vi "live view D01.vi"() -> ()   [LabVIEW 2019, in "D01.lvlib"]
uses:
  D01.lvlib
  <vilib>/userDefined/High Color/IMAQdx.ctl
  <vilib>/vision/Image Controls.llb/IMAQ Image.ctl
  <vilib>/measure/mamon.llb/Trigger Detection for 1 Channel.vi
  <vilib>/measure/NI_MAPro.lvlib
  Calibration Lib.lvlib
  database.lvlib
  <vilib>/vision/driver/NI_Vision_Acquisition_Software.lvlib
panel:
  out "Error out":errorcluster
  in  "Save Button":bool
  in  "Calib IMQ Num":u16(ring) items=["First IMQ", "Second IMQ", "Third IMQ"]
  in  "Verify Calibration1 D01":bool caption="capture grab"
  in  "snapshot":bool
  out "error prj26":errorcluster
  in  "Verify Calibration D01":bool caption="capture grab"
  in  "Close":bool
  in  "Method 2 save D01":bool caption="capture grab"
  in  "Method 1 Save D01":bool caption="Saving txt"
  out "Average Result":string="Average Result"
  out ">16  A":dbl(slide)=1.0 caption=">16 mm" scale=0.0..100.0
  out "14-16  A":dbl(slide)=1.0 caption="14.16 mm" scale=0.0..100.0
  out "12.7-14 A":dbl(slide)=1.0 caption="12.7-14 mm" scale=0.0..100.0
  out "11-12.7 A":dbl(slide)=1.0 caption="11-12.7 mm" scale=0.0..100.0
  out "9.5-11  A":dbl(slide)=1.0 caption="9.5-11 mm" scale=0.0..100.0 scale format="%#_4f"
  out "8-9.5  A":dbl(slide)=1.0 caption="8-9.5 mm" scale=0.0..100.0
  out "6.3-8  A":dbl(slide)=1.0 caption="6.3-8 mm" scale=0.0..100.0
  out "<6.3  A":dbl(slide)=1.0 caption="<6.3 mm" scale=0.0..100.0
  out "Live Result":string="Live Result"
  out ">16  L":dbl(slide)=1.0 caption=">16 mm" scale=0.0..100.0
  out "Live View":T1(plugin-control) caption="Disc 26"
  out "14-16  L":dbl(slide)=1.0 caption="14-16 mm" scale=0.0..100.0
  out "12.7-14  L":dbl(slide)=1.0 caption="12.7-14 mm" scale=0.0..100.0
  out "11-12.7L":dbl(slide)=1.0 caption="11-12.7 mm" scale=0.0..100.0
  out "9.5-11  L":dbl(slide)=1.0 caption="9.5-11 mm" scale=0.0..100.0 scale format="%#_4f"
  out "8-9.5  L":dbl(slide)=1.0 caption="8-9.5 mm" scale=0.0..100.0
  out "6.3-8  L":dbl(slide)=1.0 caption="6.3-8 mm" scale=0.0..100.0
  out "<6.3  L":dbl(slide)=1.0 caption="<6.3 mm" scale=0.0..100.0
  out "disc name":string="Live Info Disc 01"
  out "dsgs":string="DSGS"
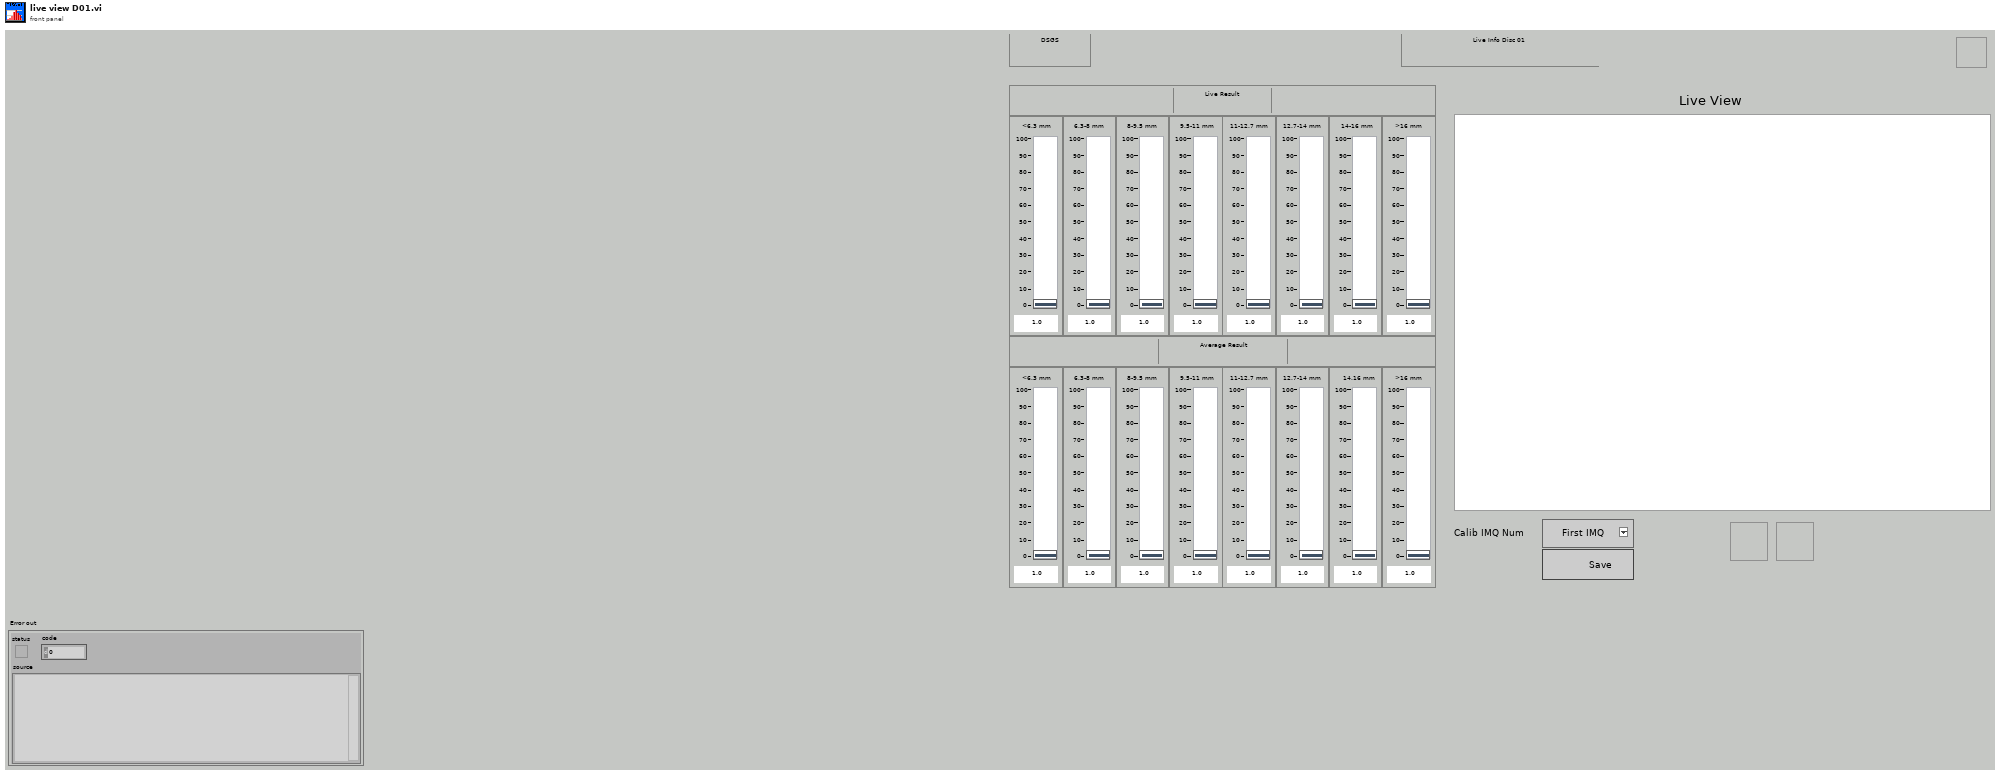
[diagram p1: front panel]
types:
  T1 = typedef "IMAQ Image.ctl" = refnum<image>
  T2 = typedef "IMAQdx.ctl" = refnum<k21>
  T3 = enum8{"Enabled", "Disabled", "Disabled and Grayed Out"}
  T4 = cluster{"date/time string":string, "date/time string":string, string, "Value":dbl, "Value":dbl, "Value":dbl, "Value":dbl, "Value":dbl, "Value":dbl, "Value":dbl, "Value":dbl}
  T5 = cluster{"date/time string":string, "date/time string":string, i32, "spreadsheet string":string, "spreadsheet string":string}
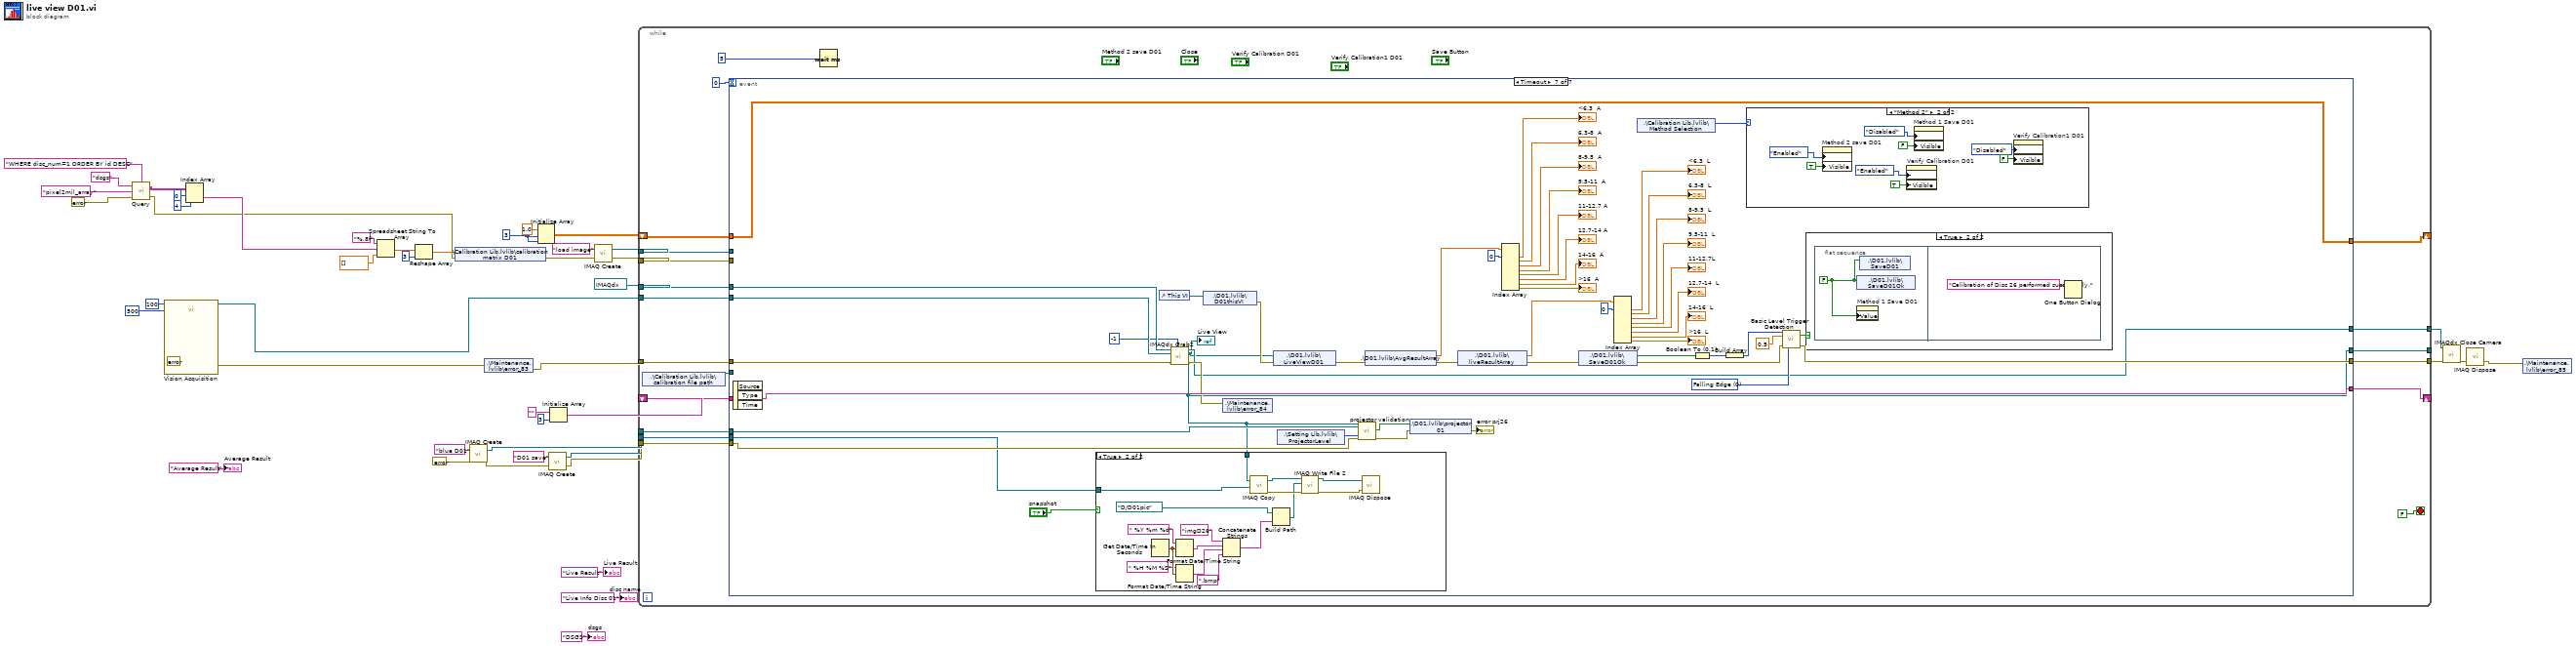
[diagram p0: block diagram]
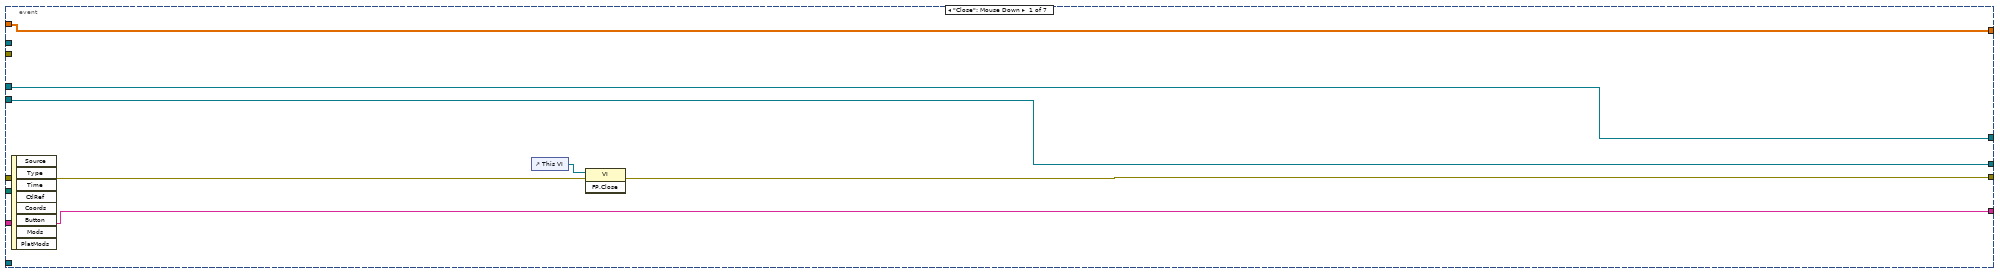
[diagram p2: hidden frame]
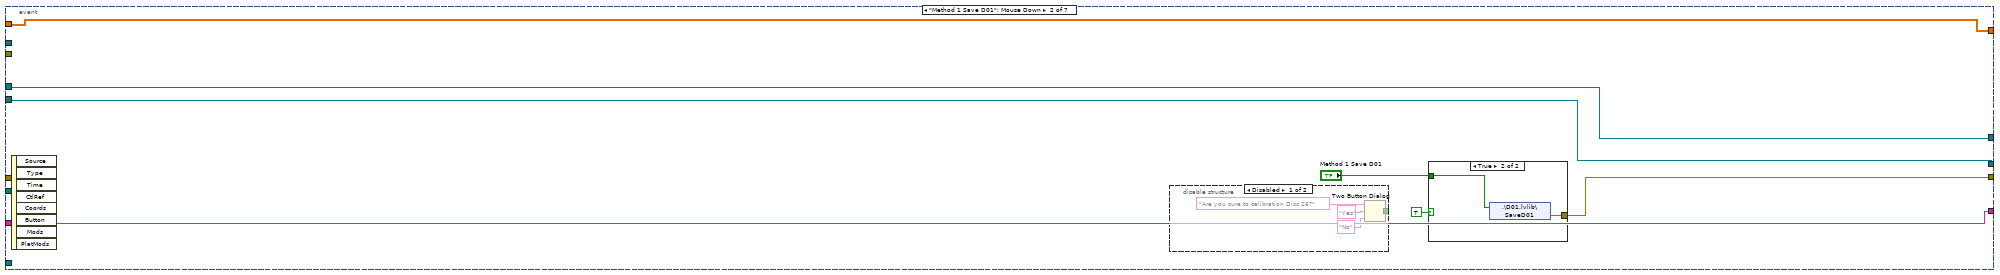
[diagram p3: hidden frame]
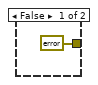
[diagram p5: hidden frame]
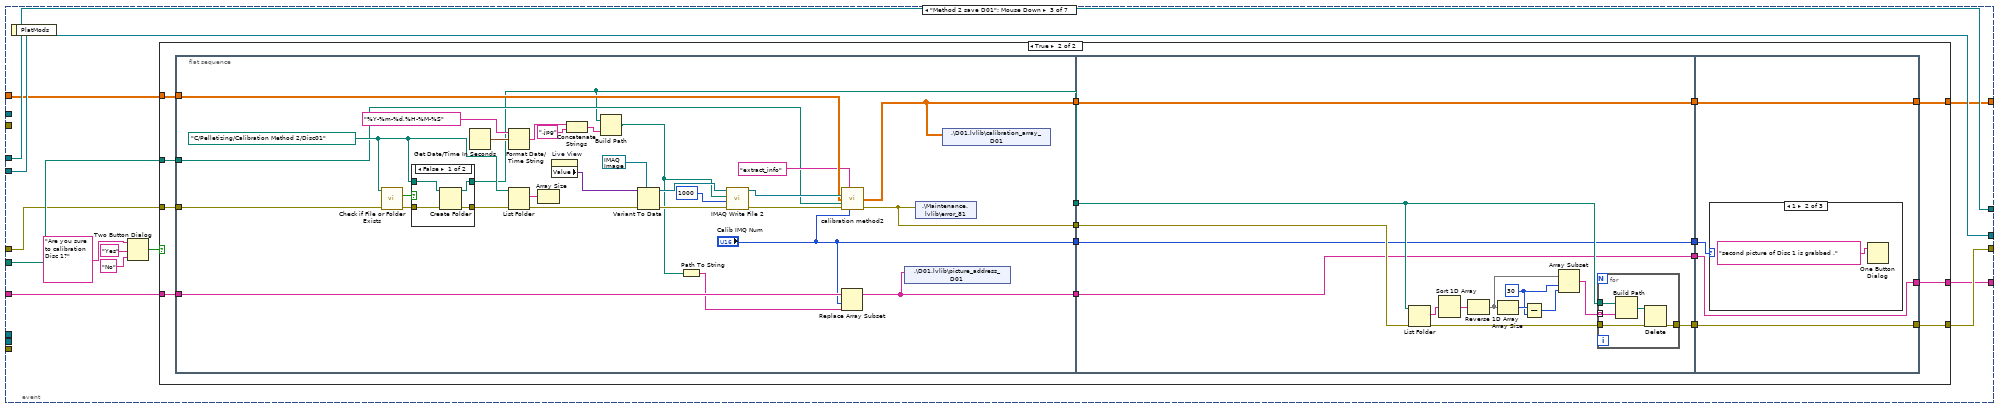
[diagram p6: hidden frame]
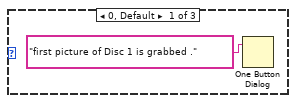
[diagram p9: hidden frame]
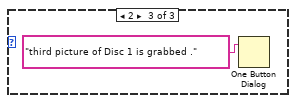
[diagram p10: hidden frame]
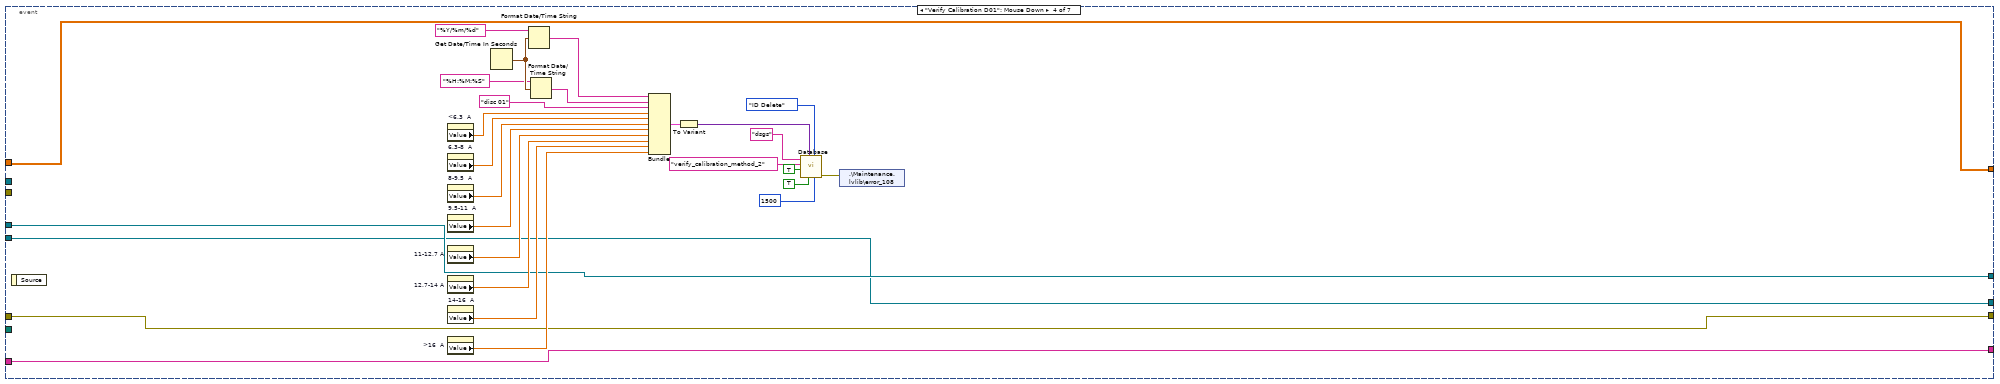
[diagram p11: hidden frame]
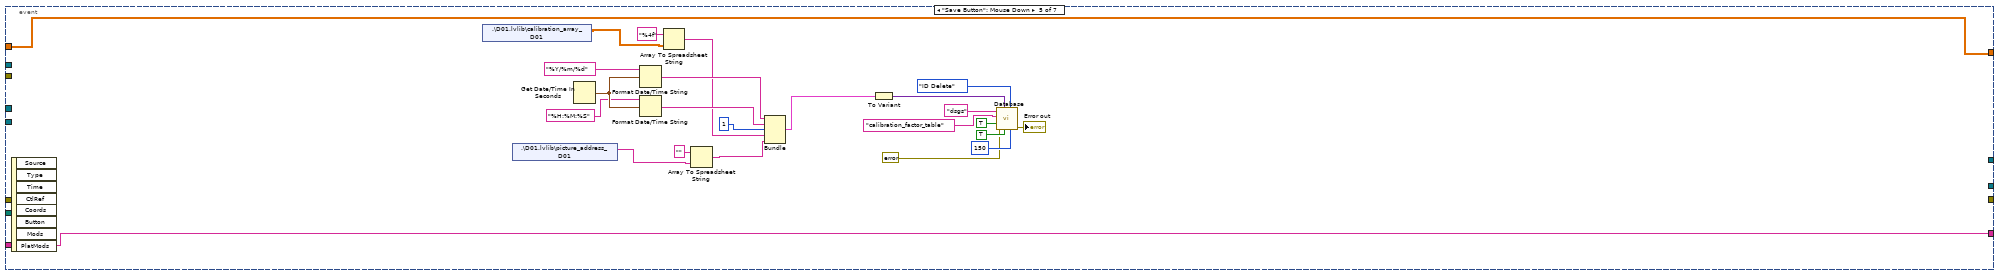
[diagram p12: hidden frame]
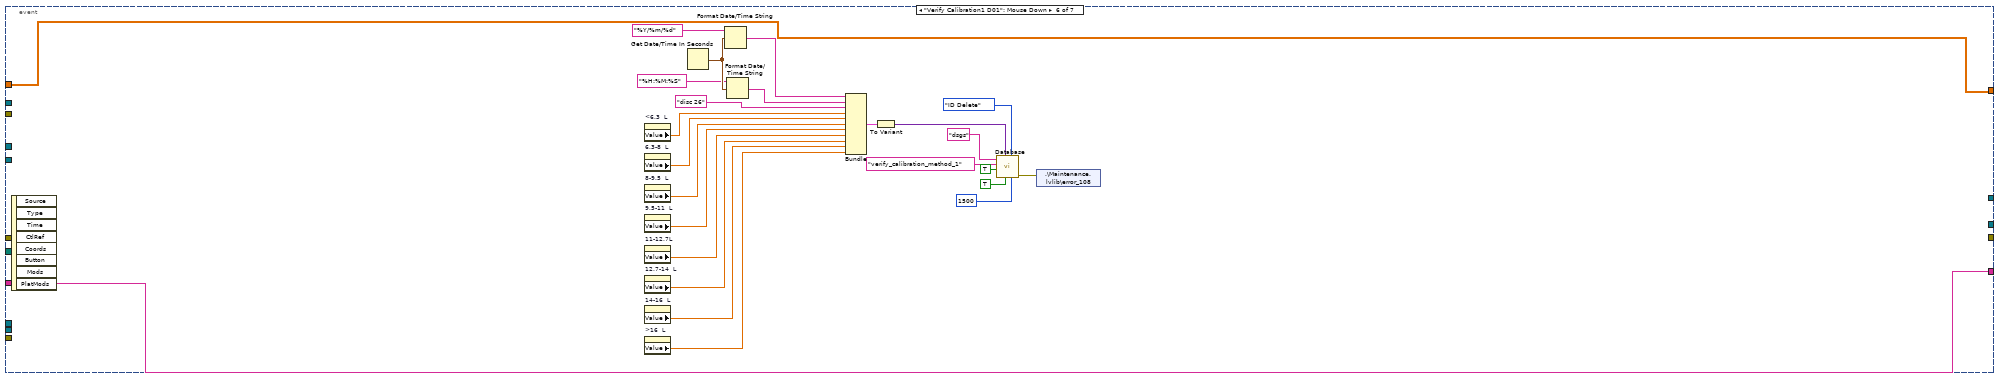
[diagram p13: hidden frame]
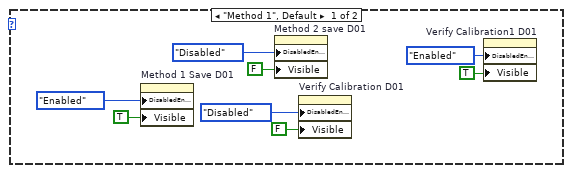
[diagram p15: hidden frame]
diagram:
  w15 = 3 ("dimension size")
  (unwired) errorcluster {"status"=FALSE, "code"=0, "source"=""} ("error in (no error)")
  n1 = call "Query.vi"("Condition"="WHERE disc_num=1 ORDER BY id DESC", "Error in"=errorcluster {"status"=FALSE, "code"=0, "source"=""}, "Table Name"="pixel2mil_array", "Connection Name"="dsgs") -> ("Error out"=w7:errorcluster, "data"=w10:string[][])
  n2 = call "Vision Acquisition"("Gain (Raw)"=i64 100, "Exposure Time (Raw)"=i64 500) -> ("Image Out"=w4:T1, "error out"=w3:errorcluster)  [unwired: 23 in, 1 out]
  n3 = Index Array(array=w10, index (row)=0, index (col)=4 ("disabled index (col)")) -> (element=w8:string)
  n4 = Spreadsheet String To Array(format string="%.8f", spreadsheet string=w8, array type (2D Dbl)=sgl[] []) -> (array=w28:sgl[])  [unwired: 1 in]
  n5 = Reshape Array(w28, 3 ("dimension size")) -> (w25:sgl[])
  n6 = shared-variable ".\\Calibration Lib.lvlib\\calibration matrix D01"(w25, error in=w7) -> (error out=w24:errorcluster)
  n7 = call "IMAQ Create"("Image Name"="blue D01", "error in (no error)"=errorcluster {"status"=FALSE, "code"=0, "source"=""}) -> ("New Image"=w22:T1, "error out"=w20:errorcluster)  [unwired: 3 in]
  n8 = shared-variable ".\\Maintenance.lvlib\\error_83"(w3) -> (error out=w37:errorcluster)  [unwired: 1 in]
  n9 = Initialize Array(1.0 ("element"), w15, w15) -> (w14:dbl[][])
  n10 = call "IMAQ Create"("Image Name"="D01 save", "error in (no error)"=w20) -> ("New Image"=w17:T1, "error out"=w19:errorcluster)  [unwired: 3 in]
  n11 = Initialize Array("", 3 ("dimension size")) -> (w11:string[])
  n12 = call "IMAQ Create"("Image Name"="load image", "error in (no error)"=w24) -> ("New Image"=w34:T1, "error out"=w35:errorcluster)  [unwired: 3 in]
  n13 = while {
    tunnel: w37 -> [w62]
    tunnel: w4 -> [w60]
    tunnel: [w59] -> w41
    tunnel: [w58] -> _
    tunnel: T2 "cam0" ("Session In") -> [w57]
    tunnel: [w56] -> w38
    tunnel: w35 -> [w55]
    tunnel: w34 -> [w54]
    tunnel: w22 -> [w53]
    tunnel: w19 -> [w52]
    tunnel: w17 -> [w51]
    shift-right: [w49] -> _
    shift-left: w14 -> [w50]
    shift-right: [w47] -> _
    shift-left: w11 -> [w48]
    stop <- FALSE stop-if-true
    n14 = shared-variable ".\\Calibration Lib.lvlib\\calibration file path"() -> (w46:path)  [unwired: 1 in, 1 out]
    n15 = event shown="[6] Timeout" {
      selector: _ -> [_ _ _ _ _ _ _]
      dyn-events: _ -> [_ _ _ _ _ _ _]
      timeout: 0 -> [_ _ _ _ _ _ _]
      tunnel: w46 -> [_ _ w98 _ _ _ _]
      tunnel: [w70 w78 w94 w186 _ _ w275] -> w59
      tunnel: w62 -> [w69 _ w97 w186 _ _ w263]
      tunnel: w60 -> [w68 w77 w96 w184 _ _ w261]
      tunnel: [w68 w77 w96 w184 _ _ w257] -> w58
      tunnel: w57 -> [w67 w76 w95 w185 _ _ w260]
      tunnel: [w67 w76 w95 w185 _ _ w258] -> w56
      tunnel: w55 -> [_ _ _ _ _ _ _]
      tunnel: w54 -> [_ _ _ _ _ _ _]
      tunnel: w53 -> [_ _ _ _ _ _ w273]
      tunnel: w52 -> [_ _ _ _ _ _ w269]
      tunnel: w51 -> [_ _ _ _ _ _ w266]
      tunnel: w50 -> [w66 w73 w89 w181 w210 w233 w265]
      tunnel: [w66 w73 w88 w181 w210 w233 w265] -> w49
      tunnel: w48 -> [w65 w72 w87 w180 w209 w232 w264]
      tunnel: [w65 w72 w86 w180 w209 w232 w264] -> w47
      event "Close": Mouse Down {
        n16 = event-data() -> ()  [unwired: 1 in, 8 out]
        n17 = control-ref of="This VI"() -> (w71:refnum<vi>)
        n18 = invoke class="VI" method="FP.Close"(reference=w71, error in=w69) -> (error out=w70:errorcluster)  [unwired: 1 in, 2 out]
      }
      event "Method 1 Save D01": Mouse Down {
        n19 = event-data() -> ()  [unwired: 1 in, 8 out]
        n20 = disable-structure shown="Disabled" {
          disable-tunnel: [w79 _] -> _
          frame Disabled {
            n21 = Two Button Dialog(message="Are you sure to calibration Disc 26?", 1:"No" ("F button name (\"Cancel\")"), 2:"Yes" ("T button name (\"OK\")")) -> (T button?=w79:bool)
          }
          frame Enabled {
          }
        }
        n22 = case shown="True" TRUE {
          tunnel: [errorcluster {"status"=FALSE, "code"=0, "source"=""} ("error IO") w85] -> w78
          tunnel: "Method 1 Save D01" -> [_ w84]
          frame False {
          }
          frame True {
            n23 = shared-variable ".\\D01.lvlib\\SaveD01"(w84) -> (error out=w85:errorcluster)  [unwired: 1 in]
          }
        }
      }
      event "Method 2 save D01": Mouse Down {
        n24 = event-data() -> ()  [unwired: 1 in, 1 out]
        n25 = Two Button Dialog(message="Are you sure to calibration Disc 1?", 1:"No" ("F button name (\"Cancel\")"), 2:"Yes" ("T button name (\"OK\")")) -> (T button?=w90:bool)
        n26 = case shown="True" w90 {
          tunnel: w98 -> [_ w116]
          tunnel: w97 -> [w101 w115]
          tunnel: [w101 w114] -> w94
          tunnel: w89 -> [w100 w112]
          tunnel: [w100 w109] -> w88
          tunnel: w87 -> [w99 w108]
          tunnel: [w99 w105] -> w86
          frame False {
          }
          frame True {
            n27 = flat-sequence {
              tunnel: w115 -> [w137]
              tunnel: w116 -> [w122]
              tunnel: [w118] -> w117
              tunnel: w112 -> [w130]
              tunnel: [w129] -> w110
              tunnel: w108 -> [w126]
              tunnel: [w125] -> w106
              tunnel: [w124] -> w104
              tunnel: ["Calib IMQ Num"] -> w102
              tunnel: [w158] -> w113
              tunnel: [w156] -> w111
              tunnel: [w155] -> w107
              tunnel: [w154] -> w103
              tunnel: w102 -> [w154]
              tunnel: w104 -> [w159]
              tunnel: w106 -> [w155]
              tunnel: w110 -> [w156]
              tunnel: w117 -> [w160]
              tunnel: [w176] -> w114
              tunnel: w113 -> [w176]
              tunnel: [w175] -> w109
              tunnel: w111 -> [w175]
              tunnel: [w174] -> w105
              tunnel: w107 -> [w174]
              tunnel: w103 -> [w173]
              frame #0 {
                w133 = path "C:/Pelletizing/Calibration Method 2/Disc01" ("path")
                n28 = call <vilib>:"Check if File or Folder Exists.vi"("error in (no error)"=w137, "path"=w133) -> ("error out"=w138:errorcluster, "file or folder exists?"=w139:bool)  [unwired: 7 in, 1 out]
                n29 = case shown="False" w139 {
                  tunnel: [w149 w153] -> w118
                  tunnel: w133 -> [w151 w153]
                  tunnel: w138 -> [w150 w152]
                  tunnel: [w148 w152] -> w135
                  frame False {
                    n30 = Create Folder(path (use dialog)=w151, error in=w150) -> (created path=w149:path, error out=w148:errorcluster)  [unwired: 1 in, 1 out]
                  }
                  frame True {
                  }
                }
                n31 = Get Date/Time In Seconds() -> (seconds since 1Jan1904=w143:timestamp)
                n32 = Format Date/Time String(time format string (%c)="%Y-%m-%d,%H-%M-%S", seconds (now)=w143) -> (date/time string=w141:string)  [unwired: 1 in]
                n33 = List Folder(path=w133, error in=w135) -> (filenames=w136:string[], error out=w134:errorcluster)  [unwired: 2 in, 2 out]
                n34 = Array Size(array=w136) -> ()  [unwired: 1 out]
                n35 = property on="Live View" class="ImageControl"() -> ("Value"=w147:variant)  [unwired: 2 in, 2 out]
                n36 = Concatenate Strings(w141, ".jpg" ("string")) -> (w121:string)
                n37 = Build Path(base path=w118, name or relative path=w121) -> (appended path=w120:path)
                n38 = Variant To Data(error in=w134, type=T1 refnum ("New Image"), Variant=w147) -> (data=w131:T1, error out=w144:errorcluster)
                n39 = Path To String(path=w120) -> (string=w119:string)
                n40 = call-poly "IMAQ Write File 2"("error in (no error)"=w144, "Image Quality"=u32 1000, "File Path"=w120, "Image"=w131) -> ("error out"=w128:errorcluster, "Image Out (duplicate)"=w132:T1)  [unwired: 6 in]
                n41 = Replace Array Subset(array=w126, new element=w119, index="Calib IMQ Num") -> (w125:string[])
                n42 = call "calibration method2.vi"("function name"="extract_info", "Image IN"=w132, "initialize matrix"=w130, "module path"=w122, "error in"=w128, "snap number"="Calib IMQ Num") -> ("calibration matrix"=w129:dbl[][], "error out"=w124:errorcluster)  [unwired: 8 in]
                n43 = shared-variable ".\\D01.lvlib\\picture_address_D01"(w125) -> ()  [unwired: 1 in, 1 out]
                n44 = shared-variable ".\\Maintenance.lvlib\\error_81"(w124) -> ()  [unwired: 1 in, 1 out]
                n45 = shared-variable ".\\D01.lvlib\\calibration_array_D01"(w129) -> ()  [unwired: 1 in, 1 out]
              }
              frame #1 {
                w161 = 30 ("index")
                n46 = List Folder(path=w160, error in=w159) -> (filenames=w167:string[], error out=w157:errorcluster)  [unwired: 2 in, 2 out]
                n47 = Sort 1D Array(array=w167) -> (sorted array=w166:string[])
                n48 = Reverse 1D Array(array=w166) -> (reversed array=w165:string[])
                n49 = Array Size(array=w165) -> (size(s)=w164:i32)
                n50 = Subtract(x=w164, y=w161) -> (x-y=w163:i32)
                n51 = Array Subset(array=w165, index=w161, length=w163) -> (w162:string[])
                n52 = for {
                  tunnel: w162 -> [w171] mode=indexing
                  tunnel: w160 -> [w172]
                  tunnel: [w169] -> w158
                  tunnel: w157 -> [w168]
                  n53 = Build Path(base path=w172, name or relative path=w171) -> (appended path=w170:path)
                  n54 = Delete(path (use dialog)=w170, error in=w168) -> (error out=w169:errorcluster)  [unwired: 3 in, 2 out]
                }
              }
              frame #2 {
                n55 = case shown="1" w173 {
                  frame 0, Default {
                    n56 = One Button Dialog(message="first picture of Disc 1 is grabbed .") -> ()  [unwired: 1 in, 1 out]
                  }
                  frame 1 {
                    n57 = One Button Dialog(message="second picture of Disc 1 is grabbed .") -> ()  [unwired: 1 in, 1 out]
                  }
                  frame 2 {
                    n58 = One Button Dialog(message="third picture of Disc 1 is grabbed .") -> ()  [unwired: 1 in, 1 out]
                  }
                }
              }
            }
          }
        }
      }
      event "Verify Calibration D01": Mouse Down {
        n59 = event-data() -> ()  [unwired: 1 in, 1 out]
        n60 = property on="<6.3  A" class="Slide (strict)"() -> ("Value"=w201:dbl)  [unwired: 2 in, 2 out]
        n61 = property on="6.3-8  A" class="Slide (strict)"() -> ("Value"=w200:dbl)  [unwired: 2 in, 2 out]
        n62 = property on="8-9.5  A" class="Slide (strict)"() -> ("Value"=w199:dbl)  [unwired: 2 in, 2 out]
        n63 = property on="9.5-11  A" class="Slide (strict)"() -> ("Value"=w198:dbl)  [unwired: 2 in, 2 out]
        n64 = property on="11-12.7 A" class="Slide (strict)"() -> ("Value"=w197:dbl)  [unwired: 2 in, 2 out]
        n65 = property on="12.7-14 A" class="Slide (strict)"() -> ("Value"=w196:dbl)  [unwired: 2 in, 2 out]
        n66 = property on="14-16  A" class="Slide (strict)"() -> ("Value"=w195:dbl)  [unwired: 2 in, 2 out]
        n67 = property on=">16  A" class="Slide (strict)"() -> ("Value"=w194:dbl)  [unwired: 2 in, 2 out]
        n68 = Get Date/Time In Seconds() -> (seconds since 1Jan1904=w206:timestamp)
        n69 = Format Date/Time String(time format string (%c)="%Y/%m/%d", seconds (now)=w206) -> (date/time string=w204:string)  [unwired: 1 in]
        n70 = Format Date/Time String(time format string (%c)="%H:%M:%S", seconds (now)=w206) -> (date/time string=w203:string)  [unwired: 1 in]
        n71 = Bundle("date/time string"=w204, "date/time string"=w203, "disc 01", "Value"=w201, "Value"=w200, "Value"=w199, "Value"=w198, "Value"=w197, "Value"=w196, "Value"=w195, "Value"=w194) -> (w193:T4)  [unwired: 1 in]
        n72 = To Variant(anything=w193) -> (Variant=w192:variant)
        n73 = call "Database.vi"("Maximum Row"=1500, "Enum"=enum16{"ID Delete", "Time Delete"}."ID Delete", "Delete row?"=TRUE, "Data"=w192, "Auto Increment ID?"=TRUE, "Table"="verify_calibration_method_2", "Connection"="dsgs") -> ("Error out"=w187:errorcluster)  [unwired: 4 in]
        n74 = shared-variable ".\\Maintenance.lvlib\\error_108"(w187) -> ()  [unwired: 1 in, 1 out]
      }
      event "Save Button": Mouse Down {
        n75 = event-data() -> ()  [unwired: 1 in, 8 out]
        n76 = shared-variable ".\\D01.lvlib\\calibration_array_D01"() -> (w211:dbl[][])  [unwired: 1 in, 1 out]
        n77 = shared-variable ".\\D01.lvlib\\picture_address_D01"() -> (w213:string[])  [unwired: 1 in, 1 out]
        n78 = Get Date/Time In Seconds() -> (seconds since 1Jan1904=w220:timestamp)
        n79 = Format Date/Time String(time format string (%c)="%Y/%m/%d", seconds (now)=w220) -> (date/time string=w221:string)  [unwired: 1 in]
        n80 = Format Date/Time String(time format string (%c)="%H:%M:%S", seconds (now)=w220) -> (date/time string=w219:string)  [unwired: 1 in]
        n81 = Array To Spreadsheet String(array=w211, 3:"%4f" ("format string")) -> (spreadsheet string=w215:string)  [unwired: 1 in]
        n82 = Array To Spreadsheet String(array=w213, 3:"" ("format string")) -> (spreadsheet string=w212:string)  [unwired: 1 in]
        n83 = Bundle("date/time string"=w221, "date/time string"=w219, 1, "spreadsheet string"=w215, "spreadsheet string"=w212) -> (w224:T5)  [unwired: 1 in]
        n84 = To Variant(anything=w224) -> (Variant=w231:variant)
        n85 = call "Database.vi"("Maximum Row"=150, "Enum"=enum16{"ID Delete", "Time Delete"}."ID Delete", "Delete row?"=TRUE, "Data"=w231, "Error in"=errorcluster {"status"=FALSE, "code"=0, "source"=""}, "Auto Increment ID?"=TRUE, "Table"="calibration_factor_table", "Connection"="dsgs") -> ("Error out"=→"Error out":errorcluster)  [unwired: 3 in]
      }
      event "Verify Calibration1 D01": Mouse Down {
        n86 = event-data() -> ()  [unwired: 1 in, 8 out]
        n87 = property on="<6.3  L" class="Slide (strict)"() -> ("Value"=w250:dbl)  [unwired: 2 in, 2 out]
        n88 = property on="6.3-8  L" class="Slide (strict)"() -> ("Value"=w249:dbl)  [unwired: 2 in, 2 out]
        n89 = property on="8-9.5  L" class="Slide (strict)"() -> ("Value"=w248:dbl)  [unwired: 2 in, 2 out]
        n90 = property on="9.5-11  L" class="Slide (strict)"() -> ("Value"=w247:dbl)  [unwired: 2 in, 2 out]
        n91 = property on="11-12.7L" class="Slide (strict)"() -> ("Value"=w246:dbl)  [unwired: 2 in, 2 out]
        n92 = property on="12.7-14  L" class="Slide (strict)"() -> ("Value"=w245:dbl)  [unwired: 2 in, 2 out]
        n93 = property on="14-16  L" class="Slide (strict)"() -> ("Value"=w244:dbl)  [unwired: 2 in, 2 out]
        n94 = property on=">16  L" class="Slide (strict)"() -> ("Value"=w243:dbl)  [unwired: 2 in, 2 out]
        n95 = Get Date/Time In Seconds() -> (seconds since 1Jan1904=w255:timestamp)
        n96 = Format Date/Time String(time format string (%c)="%Y/%m/%d", seconds (now)=w255) -> (date/time string=w253:string)  [unwired: 1 in]
        n97 = Format Date/Time String(time format string (%c)="%H:%M:%S", seconds (now)=w255) -> (date/time string=w252:string)  [unwired: 1 in]
        n98 = Bundle("date/time string"=w253, "date/time string"=w252, "disc 26", "Value"=w250, "Value"=w249, "Value"=w248, "Value"=w247, "Value"=w246, "Value"=w245, "Value"=w244, "Value"=w243) -> (w242:T4)  [unwired: 1 in]
        n99 = To Variant(anything=w242) -> (Variant=w241:variant)
        n100 = call "Database.vi"("Maximum Row"=1500, "Enum"=enum16{"ID Delete", "Time Delete"}."ID Delete", "Delete row?"=TRUE, "Data"=w241, "Auto Increment ID?"=TRUE, "Table"="verify_calibration_method_1", "Connection"="dsgs") -> ("Error out"=w236:errorcluster)  [unwired: 4 in]
        n101 = shared-variable ".\\Maintenance.lvlib\\error_108"(w236) -> ()  [unwired: 1 in, 1 out]
      }
      event Timeout {
        w283 = u16 0 items=["Falling Edge", "Rising Edge"] ("trigger slope")
        n102 = event-data() -> ()  [unwired: 1 in, 3 out]
        n103 = control-ref of="This VI"() -> (w278:refnum<vi>)
        n104 = call <vilib>:"IMAQdx Grab2.vi"("Timeout (ms)"=-1, "error in"=w263, "Image In"=w261, "Session In"=w260) -> ("error out"=w262:errorcluster, "Image Out"=w257:T1, "Session Out"=w258:T2)  [unwired: 4 in, 1 out]
        "Live View" <- w257
        n105 = case shown="True" "snapshot" {
          tunnel: w266 -> [_ w323]
          tunnel: w257 -> [_ w322]
          frame False {
          }
          frame True {
            n106 = Get Date/Time In Seconds() -> (seconds since 1Jan1904=w316:timestamp)
            n107 = Format Date/Time String(time format string (%c)=" %Y %m %d", seconds (now)=w316) -> (date/time string=w312:string)  [unwired: 1 in]
            n108 = Format Date/Time String(time format string (%c)=" %H %M %S", seconds (now)=w316) -> (date/time string=w311:string)  [unwired: 1 in]
            n109 = Concatenate Strings("imgD26" ("string"), w312, w311, ".bmp" ("string")) -> (w309:string)
            n110 = call "IMAQ Copy"("Image Dst"=w323, "Image Src"=w322) -> ("error out"=w320:errorcluster, "Image Dst Out"=w321:T1)  [unwired: 4 in]
            n111 = Build Path(base path=path "D:/D01pic" ("File Path"), name or relative path=w309) -> (appended path=w308:path)
            n112 = call-poly "IMAQ Write File 2"("error in (no error)"=w320, "File Path"=w308, "Image"=w321) -> ("error out"=w318:errorcluster, "Image Out (duplicate)"=w319:T1)  [unwired: 7 in]
            n113 = call "IMAQ Dispose"("Image"=w319, "error in (no error)"=w318) -> ()  [unwired: 4 in, 1 out]
          }
        }
        n114 = shared-variable ".\\D01.lvlib\\D01thisVI"(w278) -> (error out=w274:errorcluster)  [unwired: 1 in]
        n115 = shared-variable ".\\Maintenance.lvlib\\error_84"(w262) -> ()  [unwired: 1 in, 1 out]
        n116 = shared-variable ".\\D01.lvlib\\LiveViewD01"(w257, error in=w274) -> (error out=w277:errorcluster)
        n117 = shared-variable ".\\Setting Lib.lvlib\\ProjectorLevel"() -> (w268:i32)  [unwired: 1 in, 1 out]
        n118 = call "projector validation.vi"("Image Src"=w257, "blue channel"=w273, "on/off level"=w268, "error in (no error)"=w269) -> ("on/off"=w272:bool, "error out"=w271:errorcluster)  [unwired: 14 in]
        n119 = shared-variable ".\\D01.lvlib\\AvgResultArray"(error in=w277) -> (w298:dbl[], error out=w280:errorcluster)
        n120 = shared-variable ".\\D01.lvlib\\projector 01"(w272, error in=w271) -> (error out=→"error prj26":errorcluster)
        n121 = shared-variable ".\\D01.lvlib\\liveResultArray"(error in=w280) -> (w297:dbl[], error out=w279:errorcluster)
        n122 = Index Array(array=w298, index #1=0 ("index")) -> (element #1=→"<6.3  A":dbl, element #2=→"6.3-8  A":dbl, element #3=→"8-9.5  A":dbl, element #4=→"9.5-11  A":dbl, element #5=→"11-12.7 A":dbl, element #6=→"12.7-14 A":dbl, element #7=→"14-16  A":dbl, element #8=→">16  A":dbl)  [unwired: 7 in]
        n123 = shared-variable ".\\D01.lvlib\\SaveD01Ok"(error in=w279) -> (w284:bool, error out=w276:errorcluster)
        n124 = Index Array(array=w297, index #1=0 ("index")) -> (element #1=→"<6.3  L":dbl, element #2=→"6.3-8  L":dbl, element #3=→"8-9.5  L":dbl, element #4=→"9.5-11  L":dbl, element #5=→"11-12.7L":dbl, element #6=→"12.7-14  L":dbl, element #7=→"14-16  L":dbl, element #8=→">16  L":dbl)  [unwired: 7 in]
        n125 = shared-variable ".\\Calibration Lib.lvlib\\Method Selection"() -> (w281:enum32{"Method 1", "Method 2"})  [unwired: 1 in, 1 out]
        n126 = Boolean To (0,1)(Boolean=w284) -> (0, 1=w287:i16)
        n127 = Build Array(w287) -> (w286:i16[])
        n128 = case shown="\"Method 2\"" w281 {
          frame "Method 1", Default {
            n129 = property on="Method 1 Save D01" class="Bool (strict)"("DisabledEnum"=T3."Enabled" ("Disabled"), "Visible"=TRUE) -> ()  [unwired: 2 in, 2 out]
            n130 = property on="Method 2 save D01" class="Bool (strict)"("DisabledEnum"=T3."Disabled" ("Disabled"), "Visible"=FALSE) -> ()  [unwired: 2 in, 2 out]
            n131 = property on="Verify Calibration D01" class="Bool (strict)"("DisabledEnum"=T3."Disabled" ("Disabled"), "Visible"=FALSE) -> ()  [unwired: 2 in, 2 out]
            n132 = property on="Verify Calibration1 D01" class="Bool (strict)"("DisabledEnum"=T3."Enabled" ("Disabled"), "Visible"=TRUE) -> ()  [unwired: 2 in, 2 out]
          }
          frame "Method 2" {
            n133 = property on="Method 2 save D01" class="Bool (strict)"("DisabledEnum"=T3."Enabled" ("Disabled"), "Visible"=TRUE) -> ()  [unwired: 2 in, 2 out]
            n134 = property on="Verify Calibration D01" class="Bool (strict)"("DisabledEnum"=T3."Enabled" ("Disabled"), "Visible"=TRUE) -> ()  [unwired: 2 in, 2 out]
            n135 = property on="Method 1 Save D01" class="Bool (strict)"("DisabledEnum"=T3."Disabled" ("Disabled"), "Visible"=FALSE) -> ()  [unwired: 2 in, 2 out]
            n136 = property on="Verify Calibration1 D01" class="Bool (strict)"("DisabledEnum"=T3."Disabled" ("Disabled"), "Visible"=FALSE) -> ()  [unwired: 2 in, 2 out]
          }
        }
        n137 = call-poly <vilib>:"Basic Level Trigger Detection.vi"("signal in"=w286, "level"=0.5, "error in (no error)"=w276, "trigger slope"=w283) -> ("trigger detected?"=w282:bool, "error out"=w275:errorcluster)  [unwired: 9 in, 1 out]
        n138 = case shown="True" w282 {
          frame False {
          }
          frame True {
            n139 = flat-sequence {
              frame #0 {
                w340 = FALSE
                n140 = shared-variable ".\\D01.lvlib\\SaveD01Ok"(w340) -> ()  [unwired: 1 in, 1 out]
                n141 = property on="Method 1 Save D01" class="Bool (strict)"("Value"=w340) -> ()  [unwired: 2 in, 2 out]
                n142 = shared-variable ".\\D01.lvlib\\SaveD01"(w340) -> ()  [unwired: 1 in, 1 out]
              }
              frame #1 {
                n143 = One Button Dialog(message="Calibration of Disc 26 performed successfully.") -> ()  [unwired: 1 in, 1 out]
              }
            }
          }
        }
      }
    }
    n144 = Wait (ms)(milliseconds to wait=u32 5) -> ()  [unwired: 1 out]
  }
  n145 = call <vilib>:"IMAQdx Close Camera.vi"("error in"=w41, "Session In"=w38) -> ("error out"=w40:errorcluster)  [unwired: 9 in]
  n146 = call "IMAQ Dispose"("error in (no error)"=w40) -> ("error out"=w5:errorcluster)  [unwired: 5 in]
  n147 = shared-variable ".\\Maintenance.lvlib\\error_85"(w5) -> ()  [unwired: 1 in, 1 out]
  "Live Result" <- "Live Result" ("Live Result")
  "Average Result" <- "Average Result" ("Average Result")
  "disc name" <- "Live Info Disc 01" ("Live Result")
  "dsgs" <- "DSGS" ("Live Result")
